vi "Configure Bandwidth.vi"(8 "error in (no error)":errorcluster, 9 "Bandwidth Limit (0: Full)":u16(ring) items=["Full", "20MHZ", "25MHZ", "200MHZ", "250MHZ", "1GHZ", "3GHZ", "4GHZ"], 10 "Channel (0: Channel 1)":u16(ring) items=["Channel 1", "Channel 2", "Channel 3", "Channel 4"], 11 "VISA resource name":refnum<visa-resource-name>) -> (0 "error out":errorcluster, 3 "VISA resource name out":refnum<visa-resource-name>)   [LabVIEW 2020, in "LeCroy Wave Series.lvlib"]
doc: "Enables or disables the bandwidth-limiting lowpass filter. The command is used to set the bandwidth individually for each channel."
uses:
  LeCroy Wave Series.lvlib
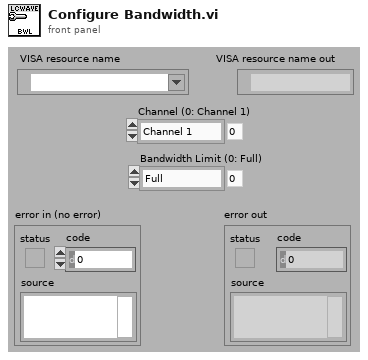
[diagram p1: front panel]
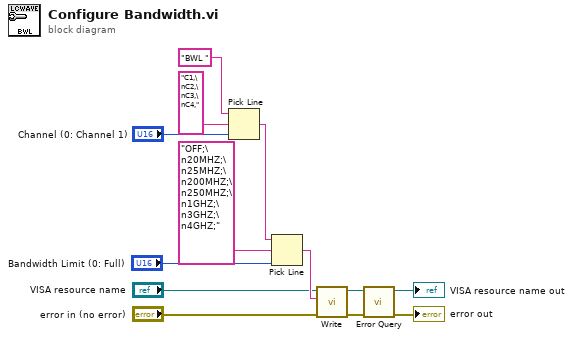
[diagram p0: block diagram]
diagram:
  n1 = Pick Line(string ("")="BWL ", multi-line string="C1,\nC2,\nC3,\nC4,", line index="Channel (0: Channel 1)") -> (output string=w8:string)
  n2 = Pick Line(string ("")=w8, multi-line string="OFF;\n20MHZ;\n25MHZ;\n200MHZ;\n250MHZ;\n1GHZ;\n3GHZ;\n4GHZ;", line index="Bandwidth Limit (0: Full)") -> (output string=w7:string)
  n3 = call "Write.vi"("error in (no error)"="error in (no error)", "Write Buffer"=w7, "VISA resource name"="VISA resource name") -> ("error out"=w1:errorcluster, "VISA resource name out"=w2:refnum<visa-resource-name>)  [unwired: 6 in, 1 out]
  n4 = call "Error Query.vi"("error in (no error)"=w1, "VISA resource name"=w2) -> ("error out"=→"error out":errorcluster, "VISA resource name out"=→"VISA resource name out":refnum<visa-resource-name>)  [unwired: 6 in, 2 out]
